vi "Cmd_U8.vi"(7 "Argument":u8 max=127 step=1, 8 "error in (no error)":errorcluster, 9 "Cmd":u8, 10 "Address":u8, 11 "VISA Refnum in":refnum<visa-resource-name>) -> (0 "error out":errorcluster, 2 "Valid":bool, 3 "VISA Refnum out":refnum<visa-resource-name>)   [LabVIEW 2015, in "Ion Motion Roboclaw.lvlib"]
uses:
  <instrlib>/Ion Motion Roboclaw/Ion Motion Roboclaw.lvlib
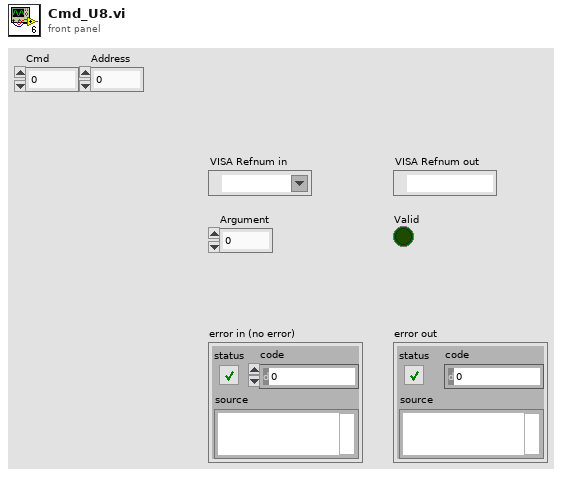
[diagram p1: front panel]
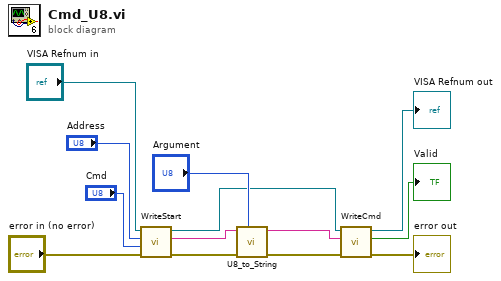
[diagram p0: block diagram]
diagram:
  n1 = call <instrlib>:"WriteStart.vi"("error in (no error)"="error in (no error)", "Cmd"="Cmd", "Address"="Address", "VISA Refnum in"="VISA Refnum in") -> ("error out"=w5:errorcluster, "String Out"=w4:string, "VISA Refnum out"=w3:refnum<visa-resource-name>)  [unwired: 5 in]
  n2 = call <instrlib>:"U8_to_String.vi"("Argument"="Argument", "error in (no error)"=w5, "String In"=w4) -> ("error out"=w9:errorcluster, "String Out"=w8:string)  [unwired: 5 in]
  n3 = call <instrlib>:"WriteCmd.vi"("error in (no error)"=w9, "write buffer"=w8, "VISA Refnum in"=w3) -> ("error out"=→"error out":errorcluster, "Valid"=→"Valid":bool, "VISA Refnum out"=→"VISA Refnum out":refnum<visa-resource-name>)  [unwired: 2 in]
